vi "Write MsgRX.vi"(8 "error in (no error)":errorcluster, 10 "MsgRX":string, 11 "Comm in":refnum<class "Comm.lvclass">) -> (0 "error out":errorcluster, 3 "Comm out":refnum<class "Comm.lvclass">)   [LabVIEW 2018, in "Comm.lvclass"]
uses:
  Comm.lvclass
  Comm.lvclass/Comm.ctl
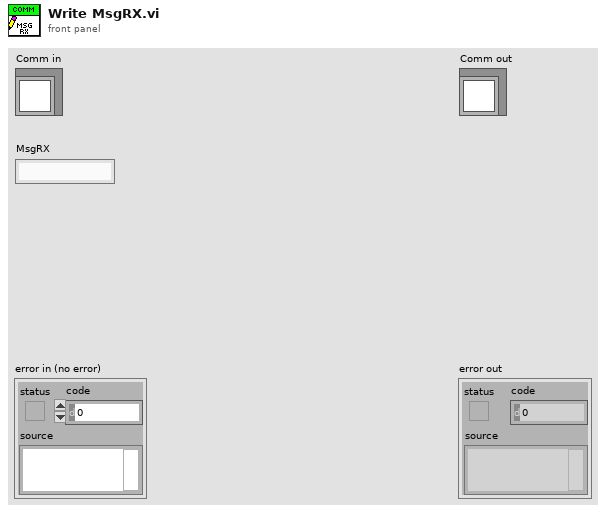
[diagram p1: front panel]
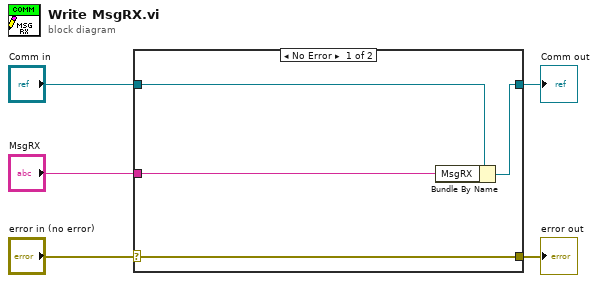
[diagram p0: block diagram]
diagram:
  n1 = case shown="No Error" "error in (no error)" {
    selector: "error in (no error)" -> [w9 w10]
    tunnel: [w9 w10] -> w4
    tunnel: [w7 w11] -> w2
    tunnel: "Comm in" -> [w8 w11]
    tunnel: "MsgRX" -> [w6 _]
    frame No Error {
      n2 = Bundle By Name(cluster=w8, "MsgRX"=w6) -> (w7:refnum<class "Comm.lvclass">)
    }
    frame Error {
    }
  }
  "error out" <- w4
  "Comm out" <- w2
